vi "Close.vi"(8 "error in (no error)":errorcluster, 11 "Local Queues":T1) -> (0 "error out":errorcluster)   [LabVIEW 2020, in "Communication VIs.lvlib" / "Local.lvlib"]
uses:
  Local.lvlib
  Local Queues.ctl
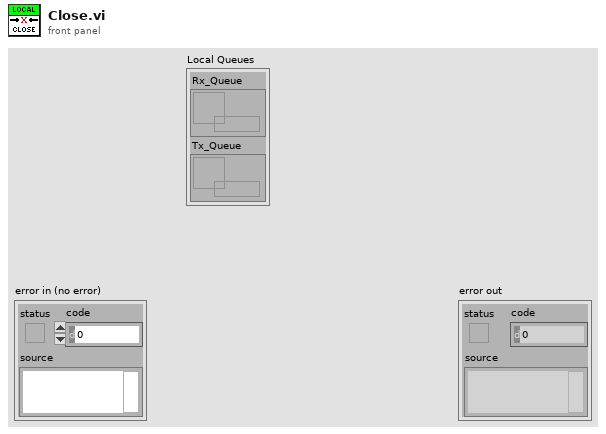
[diagram p1: front panel]
types:
  T1 = typedef "Communication VIs.lvlib/Local.lvlib/Local Queues.ctl" = cluster{"Rx_Queue":refnum<queue>, "Tx_Queue":refnum<queue>}
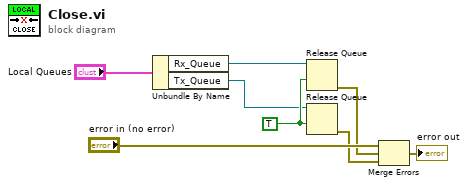
[diagram p0: block diagram]
diagram:
  w8 = TRUE
  n1 = Unbundle By Name("Local Queues") -> ("Rx_Queue"=w7:refnum<queue>, "Tx_Queue"=w6:refnum<queue>)
  n2 = Release Queue(queue=w7, force destroy? (F)=w8) -> (error out=w3:errorcluster)  [unwired: 1 in, 2 out]
  n3 = Release Queue(queue=w6, force destroy? (F)=w8) -> (error out=w2:errorcluster)  [unwired: 1 in, 2 out]
  n4 = Merge Errors("error in (no error)", w3, w2) -> (→"error out":errorcluster)
